vi "SetTrig sync en.vi"(8 "error in (no error)":errorcluster, 10 "Trig sync en":bool, 11 "reference in":refnum<class "mmWave instrument.lvclass">) -> (0 "error out":errorcluster, 3 "reference out":refnum<class "mmWave instrument.lvclass">)   [LabVIEW 2019, in "mmWave instrument.lvclass"]
uses:
  mmWave instrument.lvclass
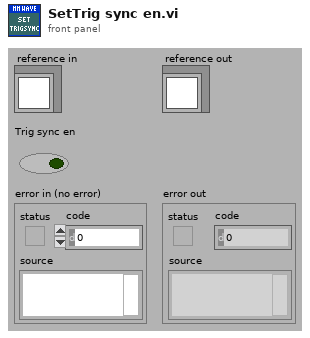
[diagram p1: front panel]
types:
  T1 = typedef "mmWave instrument.lvclass/ObjectAttributesRef.ctl" = refnum<data-value>
  T2 = typedef "mmWave instrument.lvclass/ObjectAttributes.ctl" = cluster{"mode":T3, "instr state":T4, "Max Fs":dbl, "Equalization coeff":cdb[], "LO sync en":bool, "Trig sync en":bool, "LO sources":T5, "LO Export":T6, "Fc.range":cluster{"min":dbl, "max":dbl}, "Sync mode":T7, "equalization en":bool, "sequence":string[]}
  T3 = typedef "mmWave instrument.lvclass/Instrument mode.ctl" = enum16{"RF", "IF", "BB"}
  T4 = typedef "mmWave instrument.lvclass/Instrument state.ctl" = enum16{"Off", "Initialization", "Configuration", "Running", "Calibration"}
  T5 = typedef "mmWave HW Control.lvlib/LO sources.ctl" = cluster{"RX/LO1 src":string, "TX/LO1 src":string, "LO2 src":string}
  T6 = typedef "mmWave HW Control.lvlib/LO export.ctl" = cluster{"TX LO1 export":bool, "TX LO1 export level":dbl, "RX LO1 export":bool, "RX LO1 export level":dbl, "LO2 export":bool, "LO2 export level":dbl}
  T7 = typedef "mmWave instrument.lvclass/Sync mode.ctl" = enum16{"Slave", "Master"}
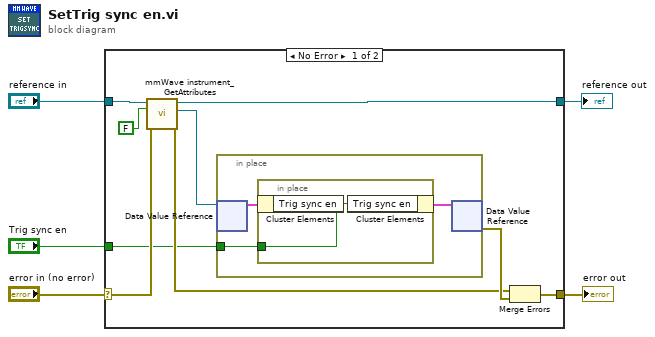
[diagram p0: block diagram]
diagram:
  n1 = case shown="No Error" "error in (no error)" {
    selector: "error in (no error)" -> [w14 w20]
    tunnel: [w8 w20] -> w4
    tunnel: [w13 w19] -> w2
    tunnel: "reference in" -> [w12 w19]
    tunnel: "Trig sync en" -> [w6 _]
    frame No Error {
      n2 = call "mmWave instrument_GetAttributes.vi"("error in (no error)"=w14, "return data? (T)"=FALSE, "reference in"=w12) -> ("error out"=w9:errorcluster, "attributes ref"=w7:T1, "reference out"=w13:refnum<class "mmWave instrument.lvclass">)  [unwired: 5 in, 1 out]
      n3 = in-place {
        in-place-border: w6 -> [w15]
        n4 = in-place-dvr #1(w7) -> (w16:T2)  [unwired: 1 out]
        n5 = in-place {
          in-place-border: w15 -> [w18]
          n6 = in-place-cluster #2(w16) -> ()  [unwired: 1 out]
          n7 = in-place-cluster #2("Trig sync en"=w18) -> (w17:T2)
        }
        n8 = in-place-dvr #1(w17) -> (w10:errorcluster)  [unwired: 1 out]
      }
      n9 = Merge Errors(w9, w10) -> (w8:errorcluster)
    }
    frame Error {
    }
  }
  "error out" <- w4
  "reference out" <- w2
